vi "MedianFilter_ResetToValue.vi"(9 "Value":dbl, 11 "In MEDIAN_FILTER":T1 {"ValueBuffer" format="%13.5g"}) -> (3 "Out MEDIAN_FILTER":T1 {"ValueBuffer" format="%13.5g"})   [LabVIEW 2019, in "Trajectory_Library.lvlib"]
doc: "Resets the filter, clearing the window of all elements. All stored values are set to \"value:\".\n\nInputs:\n - Value -- Storage buffer elements are set to this value.\n - In Median Filter -- Median filter data structure\n\nOutputs:\n - Out Median Filter -- Updated median filter data structure"
uses:
  Trajectory_Library.lvlib
  TypeDef/MEDIAN_FILTER.ctl
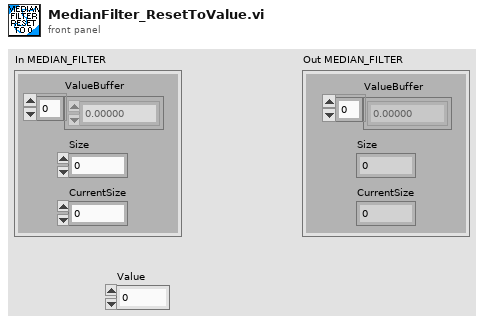
[diagram p1: front panel]
types:
  T1 = typedef "Trajectory_Library.lvlib/MEDIAN_FILTER.ctl" = cluster{"ValueBuffer":dbl[], "Size":i32, "CurrentSize":i32}
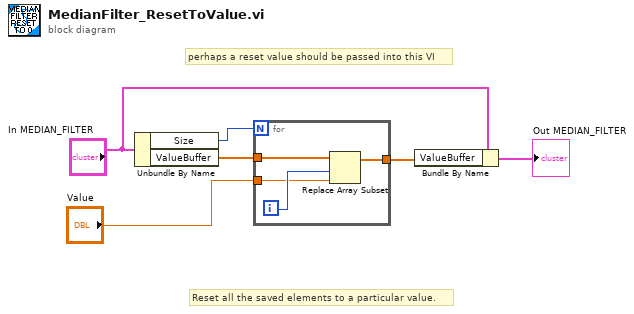
[diagram p0: block diagram]
diagram:
  # "perhaps a reset value should be passed into this VI"
  # "Reset all the saved elements to a particular value."
  n1 = Unbundle By Name("In MEDIAN_FILTER") -> ("Size"=w2:i32, "ValueBuffer"=w6:dbl[])
  n2 = for {
    N: w2 -> [_]
    tunnel: w6 -> [w10]
    tunnel: [w8] -> w5
    tunnel: "Value" -> [w7]
    i -> [w9]
    n3 = Replace Array Subset(array=w10, new element=w7, index=w9) -> (w8:dbl[])
  }
  n4 = Bundle By Name(cluster="In MEDIAN_FILTER", "ValueBuffer"=w5) -> (→"Out MEDIAN_FILTER":T1)
